vi "User32dllAPI.GetDisplays.vi"(11 "monitor":i32) -> (0 "#displays":i32, 1 "monitor height":i16, 2 "monitor width":i16, 3 "offset":i16)   [LabVIEW 2010]
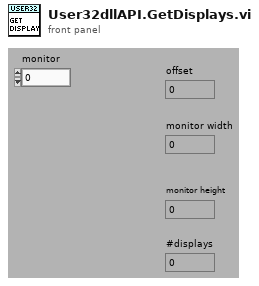
[diagram p1: front panel]
types:
  T1 = typedef "LVAllMonitorsDisplayTypeDef.ctl" = cluster{"Bounds":cluster{"Left":i16, "Top":i16, "Right":i16, "Bottom":i16}, "Depth":i16}[]
  T2 = cluster{"Bounds":cluster{"Left":i16, "Top":i16, "Right":i16, "Bottom":i16}, "Depth":i16}
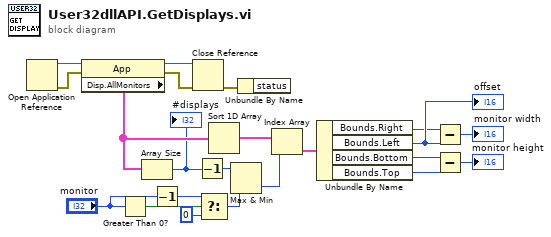
[diagram p0: block diagram]
diagram:
  n1 = Open Application Reference() -> (0:w17:errorcluster, 3:w18:refnum<vi>)  [unwired: 4 in]
  n2 = property class="App"(reference=w18, error in=w17) -> (reference out=w16:refnum<vi>, error out=w15:errorcluster, "Disp.AllMonitors"=w7:T1)
  n3 = Greater Than 0?(x="monitor") -> (x > 0?=w12:bool)
  n4 = Array Size(array=w7) -> (size(s)=w4:i32)
  "#displays" <- w4
  n5 = Decrement(x="monitor") -> (x-1=w1:i32)
  n6 = Close Reference(reference=w16, error in (no error)=w15) -> (error out=w14:errorcluster)
  n7 = Decrement(x=w4) -> (x-1=w3:i32)
  n8 = Select(t=w1, s=w12, f=0 ("t")) -> (s? t:f=w6:i32)
  n9 = Sort 1D Array(array=w7) -> (sorted array=w10:T1)
  n10 = Max & Min(x=w3, y=w6) -> (min(x,y)=w5:i32)  [unwired: 1 out]
  n11 = Unbundle By Name(w14) -> ()  [unwired: 1 out]
  n12 = Index Array(array=w10, index=w5) -> (element=w8:T2)
  n13 = Unbundle By Name(w8) -> ("Bounds.Right"=w13:i16, "Bounds.Left"=w22:i16, "Bounds.Bottom"=w11:i16, "Bounds.Top"=w9:i16)
  "offset" <- w22
  n14 = Subtract(x=w13, y=w22) -> (x-y=→"monitor width":i16)
  n15 = Subtract(x=w11, y=w9) -> (x-y=→"monitor height":i16)
